vi "Get Pattern Name.vi"(11 "Config file in":path) -> (3 "Pattern Name":string)   [LabVIEW 2018]
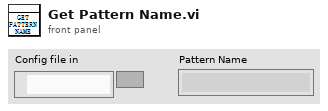
[diagram p1: front panel]
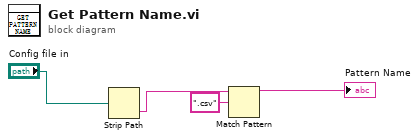
[diagram p0: block diagram]
diagram:
  n1 = Strip Path(path="Config file in") -> (name=w3:string)  [unwired: 1 out]
  n2 = Match Pattern(string=w3, regular expression=".csv") -> (before substring=→"Pattern Name":string)  [unwired: 1 in, 3 out]
